vi "GetAngle.vi"(11 "navX Device TypeDef":T1={"navX Interface Protocol"=enum."SPI", "navX Interface Protocol TypeDefs"={"SPIDevRef"={"DevStatus"={"status"=FALSE, "code"=0, "source"=""}, "Handle"=0, "Controller"=enum."Controller 1", "SPI Bus"=enum."SPI On-Board, CS0"}, "I2CDevRef"={"DevStatus"={"status"=FALSE, "code"=0, "source"=""}, "Controller"=enum."Controller 1", "Device Address"=0, "Handle"=0, "I2C Bus"=enum."Invalid"}}, "navX System Information"={"Board Information"={"WhoAmI (50 | 0x32)"=0, "Board Revision"=0, "Firmware Major Version"=0, "Firmware Minor Version"=0, "NAVX_BOARD_CAPABILITY"={"OMNIMOUNT"=FALSE, "YAW_RESET"=FALSE, "VEL_AND_DISP"=FALSE}, "NAVX_BOARD_YAW_AXIS"={"BOARD_YAW_AXIS_UP"=FALSE, "BOARD_YAW_AXIS"=0}}, "Status"={"Update Rate Hz"=0, "Accelerometer Full-Scale Range"=0, "Gyro Full-Scale Range"=0, "NAVX_OP_STATUS"=0, "NAVX_CAL_STATUS"=0, "NAVX_SELFTEST_STATUS"=0, "NAVX_SENSOR_STATUS"={"MOVING"=FALSE, "YAW_STABLE"=FALSE, "MAG_DISTURBANCE"=FALSE, "ALTITUDE_VALID"=FALSE, "SEALEVEL_PRESS_SET"=FALSE, "FUSED_HEADING_VALID"=FALSE}}, "Offsets"={"Yaw"=0.0, "Quat W"=0.0, "Quat X"=0.0, "Quat Y"=0.0, "Quat Z"=0.0}, "LastSampleTimestamp"=0.0, "LastSampleValid"=FALSE, "LastSampleValidTimestamp"=0.0}, "navX Common Information"={"Update Rate (4Hz-60Hz)"=50, "refnum name"="", "error"={"status"=FALSE, "code"=0, "source"=""}, "LastSampleFPGATimestamp"=0.0}} {"navX Common Information"."Update Rate (4Hz-60Hz)" min=4 max=60 step=1; "navX System Information"."Status"."NAVX_OP_STATUS" items=["INITIALIZING", "SELFTEST_IN_PROGRESS", "ERROR", "IMU_AUTOCAL_IN_PROGRESS", "NORMAL"]; "navX System Information"."Status"."NAVX_CAL_STATUS" items=["IMU_CAL_STATE_MASK"=3, "IMU_CAL_INPROGRESS"=0, "IMU_CAL_ACCUMULATE"=1, "IMU_CAL_COMPLETE"=2, "MAG_CAL_COMPLETE"=4, "BARO_CAL_COMPLETE"=8]; "navX Interface Protocol TypeDefs"."I2CDevRef"."Device Address" format="%.0x"}) -> (1 "Valid?":bool, 2 "ContinuousAngle":dbl, 3 "navX Device TypeDef":T1={"navX Interface Protocol"=enum."SPI", "navX Interface Protocol TypeDefs"={"SPIDevRef"={"DevStatus"={"status"=FALSE, "code"=0, "source"=""}, "Handle"=0, "Controller"=enum."Controller 1", "SPI Bus"=enum."SPI On-Board, CS0"}, "I2CDevRef"={"DevStatus"={"status"=FALSE, "code"=0, "source"=""}, "Controller"=enum."Controller 1", "Device Address"=0, "Handle"=0, "I2C Bus"=enum."Invalid"}}, "navX System Information"={"Board Information"={"WhoAmI (50 | 0x32)"=0, "Board Revision"=0, "Firmware Major Version"=0, "Firmware Minor Version"=0, "NAVX_BOARD_CAPABILITY"={"OMNIMOUNT"=FALSE, "YAW_RESET"=FALSE, "VEL_AND_DISP"=FALSE}, "NAVX_BOARD_YAW_AXIS"={"BOARD_YAW_AXIS_UP"=FALSE, "BOARD_YAW_AXIS"=0}}, "Status"={"Update Rate Hz"=0, "Accelerometer Full-Scale Range"=0, "Gyro Full-Scale Range"=0, "NAVX_OP_STATUS"=0, "NAVX_CAL_STATUS"=0, "NAVX_SELFTEST_STATUS"=0, "NAVX_SENSOR_STATUS"={"MOVING"=FALSE, "YAW_STABLE"=FALSE, "MAG_DISTURBANCE"=FALSE, "ALTITUDE_VALID"=FALSE, "SEALEVEL_PRESS_SET"=FALSE, "FUSED_HEADING_VALID"=FALSE}}, "Offsets"={"Yaw"=0.0, "Quat W"=0.0, "Quat X"=0.0, "Quat Y"=0.0, "Quat Z"=0.0}, "LastSampleTimestamp"=0.0, "LastSampleValid"=FALSE, "LastSampleValidTimestamp"=0.0}, "navX Common Information"={"Update Rate (4Hz-60Hz)"=50, "refnum name"="", "error"={"status"=FALSE, "code"=0, "source"=""}, "LastSampleFPGATimestamp"=0.0}} {"navX Common Information"."Update Rate (4Hz-60Hz)" min=4 max=60 step=1; "navX System Information"."Status"."NAVX_OP_STATUS" items=["INITIALIZING", "SELFTEST_IN_PROGRESS", "ERROR", "IMU_AUTOCAL_IN_PROGRESS", "NORMAL"]; "navX System Information"."Status"."NAVX_CAL_STATUS" items=["IMU_CAL_STATE_MASK"=3, "IMU_CAL_INPROGRESS"=0, "IMU_CAL_ACCUMULATE"=1, "IMU_CAL_COMPLETE"=2, "MAG_CAL_COMPLETE"=4, "BARO_CAL_COMPLETE"=8]; "navX Interface Protocol TypeDefs"."I2CDevRef"."Device Address" format="%.0x"})   [LabVIEW 2014, in "navX-MXP IMU.lvlib"]
doc: "Returns the angle, in degrees, from the original heading that the robot is currently facing.\n\nNote that this angle is continuous (meaning that it can return values greater than 360 degrees and less than -360 degrees. You can devide by 360 and use the remainder to yield an angle with a value from -360 to 360 degrees.\n\nThis VI is created to provide an interface which is compatible with the WPI LabVIEW Library GetAngle.vi ."
uses:
  navX-MXP IMU.lvlib
  TypeDefs/navX Device TypeDef.ctl
  TypeDefs/Value TypeDefs/navX Interface Protocol.ctl
  <vilib>/Rock Robotics/WPI/SPI/WPI_SPIDevRef.ctl
  <vilib>/Rock Robotics/SystemInterfaces/Typedef/FPGA_TypedefDigitalModule.ctl
  <vilib>/Rock Robotics/SystemInterfaces/spilib/spi_bus.ctl
  <vilib>/Rock Robotics/WPI/I2C/WPI_I2CDevRef.ctl
  <vilib>/Rock Robotics/SystemInterfaces/i2clib/i2c_bus.ctl
  TypeDefs/Data TypeDefs/navX Board Information.ctl
  TypeDefs/Value TypeDefs/navX NAVX_BOARD_CAPABILITY.ctl
  TypeDefs/Value TypeDefs/navX NAVX_BOARD_YAW_AXIS.ctl
  TypeDefs/Data TypeDefs/navX Status Data.ctl
  TypeDefs/Value TypeDefs/navX NAVX_OP_STATUS.ctl
  TypeDefs/Value TypeDefs/navX NAVX_CAL_STATUS.ctl
  TypeDefs/Value TypeDefs/navX NAVX_SENSOR_STATUS.ctl
  TypeDefs/Data TypeDefs/navX Offsets Data.ctl
  TypeDefs/Value TypeDefs/navX Update Rate.ctl
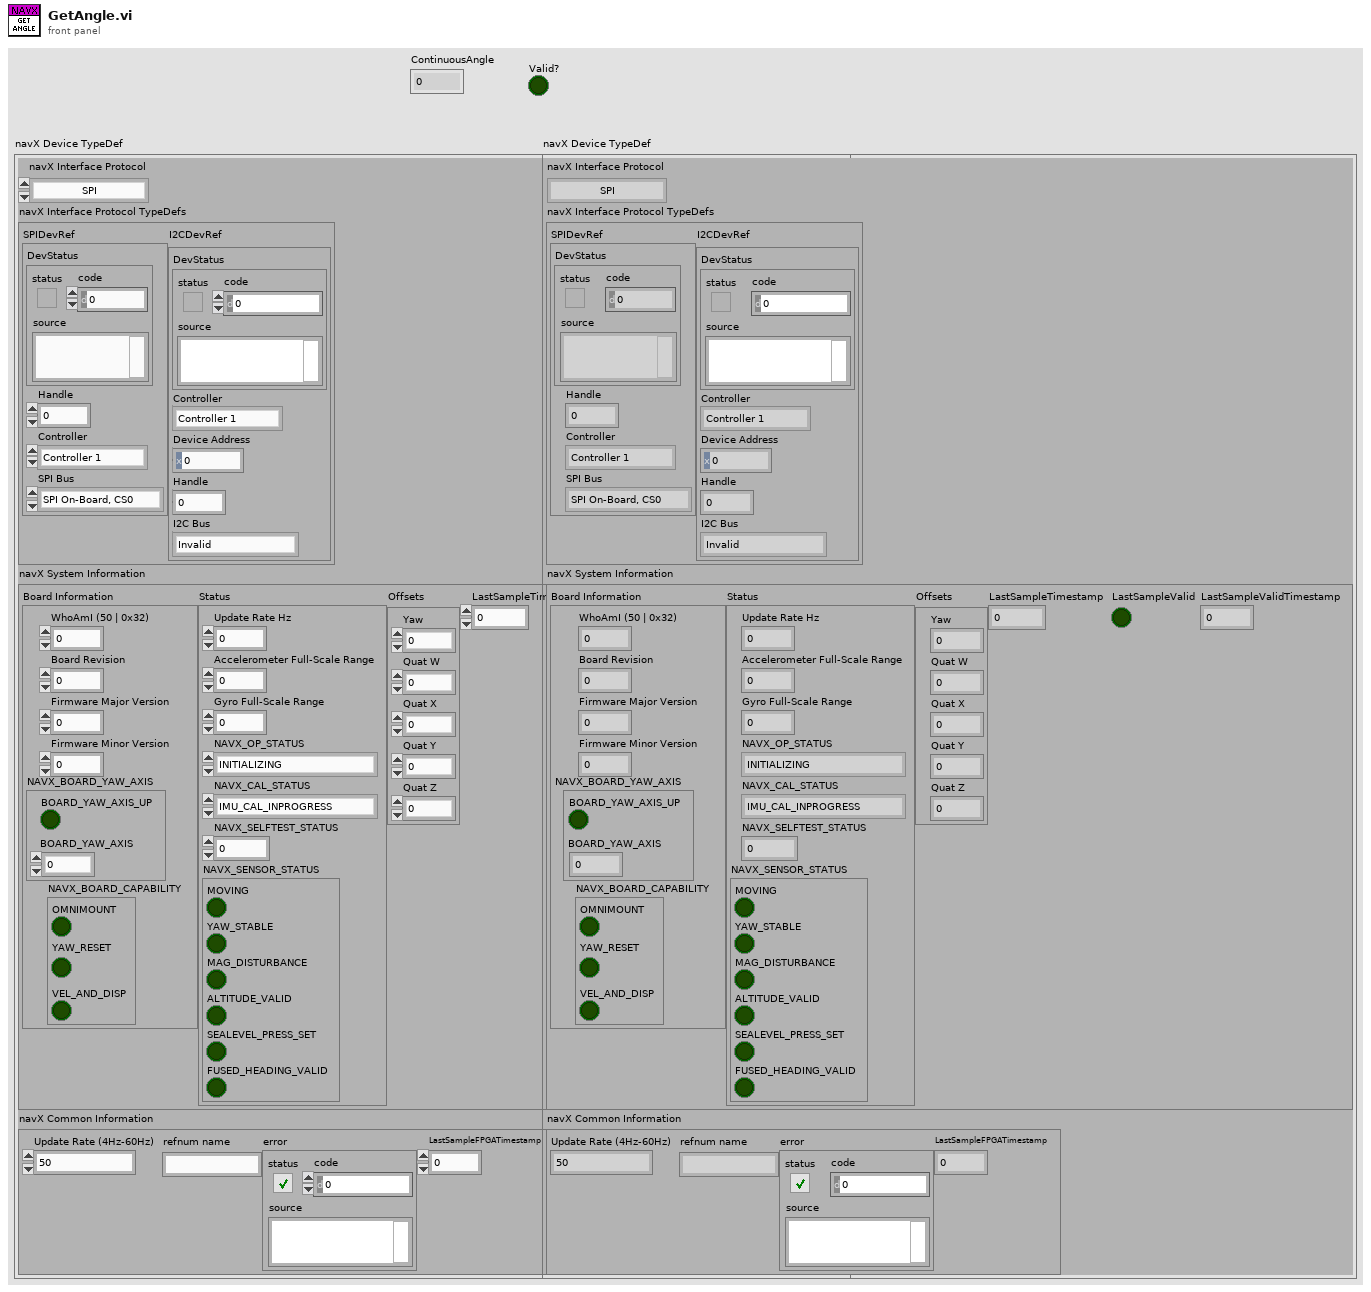
[diagram p1: front panel]
types:
  T1 = typedef "navX-MXP IMU.lvlib/navX Device TypeDef.ctl" = cluster{"navX Interface Protocol":T2, "navX Interface Protocol TypeDefs":cluster{"SPIDevRef":T3, "I2CDevRef":T6}, "navX System Information":cluster{"Board Information":T8, "Status":T11, "Offsets":T15, "LastSampleTimestamp":dbl, "LastSampleValid":bool, "LastSampleValidTimestamp":dbl}, "navX Common Information":cluster{"Update Rate (4Hz-60Hz)":T16, "refnum name":string, "error":errorcluster, "LastSampleFPGATimestamp":dbl}}
  T2 = typedef "navX-MXP IMU.lvlib/navX Interface Protocol.ctl" = enum16{"SPI", "I2C", "SERIAL"}
  T3 = typedef "WPI_SPIDevRef.ctl" = cluster{"DevStatus":errorcluster, "Handle":i32, "Controller":T4, "SPI Bus":T5}
  T4 = typedef "FPGA_TypedefDigitalModule.ctl" = enum16{"Controller 1"}
  T5 = typedef "spi_bus.ctl" = enum16{"SPI On-Board, CS0", "SPI On-Board, CS1", "SPI On-Board, CS2", "SPI On-Board, CS3", "SPI MXP", "Invalid"}
  T6 = typedef "WPI_I2CDevRef.ctl" = cluster{"DevStatus":errorcluster, "Controller":T4, "Device Address":u8, "Handle":i32, "I2C Bus":T7}
  T7 = typedef "i2c_bus.ctl" = enum16{"I2C On-Board", "I2C MXP", "Invalid"}
  T8 = typedef "navX-MXP IMU.lvlib/navX Board Information.ctl" = cluster{"WhoAmI (50 | 0x32)":u8, "Board Revision":u8, "Firmware Major Version":u8, "Firmware Minor Version":u8, "NAVX_BOARD_CAPABILITY":T9, "NAVX_BOARD_YAW_AXIS":T10}
  T9 = typedef "navX-MXP IMU.lvlib/navX NAVX_BOARD_CAPABILITY.ctl" = cluster{"OMNIMOUNT":bool, "YAW_RESET":bool, "VEL_AND_DISP":bool}
  T10 = typedef "navX-MXP IMU.lvlib/navX NAVX_BOARD_YAW_AXIS.ctl" = cluster{"BOARD_YAW_AXIS_UP":bool, "BOARD_YAW_AXIS":u8}
  T11 = typedef "navX-MXP IMU.lvlib/navX Status Data.ctl" = cluster{"Update Rate Hz":u8, "Accelerometer Full-Scale Range":u8, "Gyro Full-Scale Range":u16, "NAVX_OP_STATUS":T12, "NAVX_CAL_STATUS":T13, "NAVX_SELFTEST_STATUS":u8, "NAVX_SENSOR_STATUS":T14}
  T12 = typedef "navX-MXP IMU.lvlib/navX NAVX_OP_STATUS.ctl" = u8
  T13 = typedef "navX-MXP IMU.lvlib/navX NAVX_CAL_STATUS.ctl" = u8
  T14 = typedef "navX-MXP IMU.lvlib/navX NAVX_SENSOR_STATUS.ctl" = cluster{"MOVING":bool, "YAW_STABLE":bool, "MAG_DISTURBANCE":bool, "ALTITUDE_VALID":bool, "SEALEVEL_PRESS_SET":bool, "FUSED_HEADING_VALID":bool}
  T15 = typedef "navX-MXP IMU.lvlib/navX Offsets Data.ctl" = cluster{"Yaw":dbl, "Quat W":dbl, "Quat X":dbl, "Quat Y":dbl, "Quat Z":dbl}
  T16 = typedef "navX-MXP IMU.lvlib/navX Update Rate.ctl" = u8
  T17 = typedef "navX-MXP IMU.lvlib/navX YPRH Data.ctl" = cluster{"Yaw":dbl, "Pitch":dbl, "Roll":dbl, "Heading":dbl}
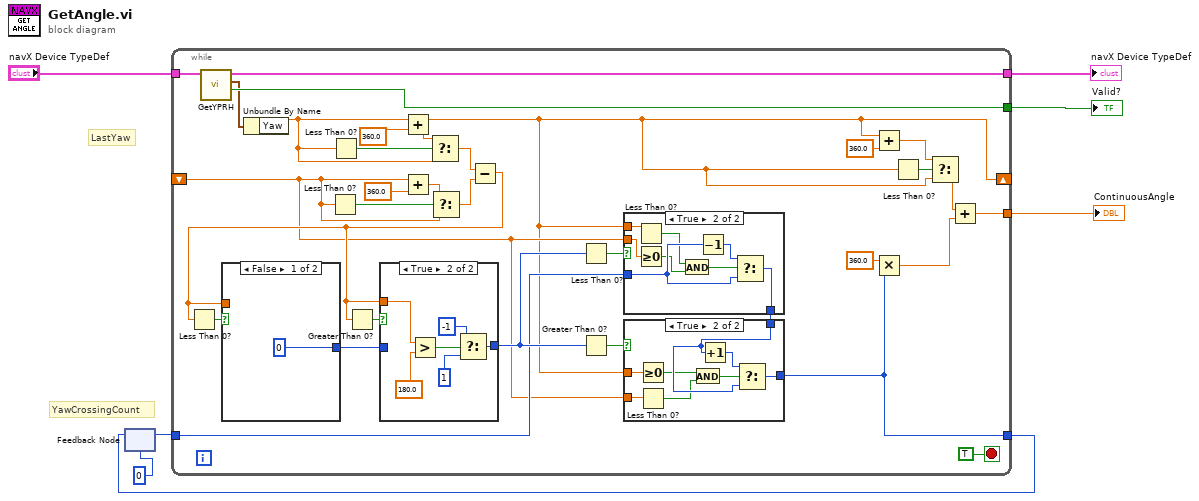
[diagram p0: block diagram]
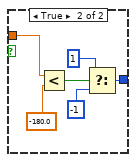
[diagram p5: hidden frame]
diagram:
  # "YawCrossingCount"
  # "LastYaw"
  n1 = feedback #1(0) -> (w3:i32)
  n2 = while {
    shift-right: [w9] -> _
    shift-left: _ -> [w10]
    tunnel: [w38] -> w5
    tunnel: "navX Device TypeDef" -> [w35]
    tunnel: [w34] -> w6
    tunnel: [w24] -> w4
    tunnel: w3 -> [w22]
    tunnel: [w21] -> w1
    stop <- TRUE stop-if-true
    n3 = call "GetYPRH.vi"("navX Device TypeDef"=w35) -> ("Valid?"=w38:bool, "YPRH"=w33:T17, "navX Device TypeDef"=w34:T1)  [unwired: 8 in]
    n4 = Unbundle By Name(w33) -> ("Yaw"=w9:dbl)
    n5 = Less Than 0?(x=w10) -> (x < 0?=w14:bool)
    n6 = Less Than 0?(x=w9) -> (x < 0?=w15:bool)
    n7 = Add(x=w9, y=360.0) -> (x+y=w8:dbl)
    n8 = Add(x=w10, y=360.0) -> (x+y=w11:dbl)
    n9 = Select(t=w8, s=w15, f=w9) -> (s? t:f=w13:dbl)
    n10 = Select(t=w11, s=w14, f=w10) -> (s? t:f=w12:dbl)
    n11 = Subtract(x=w13, y=w12) -> (x-y=w16:dbl)
    n12 = Less Than 0?(x=w16) -> (x < 0?=w18:bool)
    n13 = case shown="False" w18 {
      tunnel: [0 w67] -> w32
      tunnel: w16 -> [_ w66]
      frame False {
      }
      frame True {
        n14 = Less?(x=w66, y=-180.0) -> (x < y?=w70:bool)
        n15 = Select(t=1, s=w70, f=-1) -> (s? t:f=w67:i32)
      }
    }
    n16 = Greater Than 0?(x=w16) -> (x > 0?=w17:bool)
    n17 = case shown="True" w17 {
      tunnel: [w58 w60] -> w29
      tunnel: w32 -> [w58 _]
      tunnel: w16 -> [_ w59]
      frame False {
      }
      frame True {
        n18 = Greater?(x=w59, y=180.0) -> (0:w63:bool)
        n19 = Select(t=-1, s=w63, f=1) -> (s? t:f=w60:i32)
      }
    }
    n20 = Less Than 0?(x=w29) -> (x < 0?=w31:bool)
    n21 = Greater Than 0?(x=w29) -> (x > 0?=w30:bool)
    n22 = case shown="True" w31 {
      tunnel: w22 -> [w49 w56]
      tunnel: w9 -> [_ w54]
      tunnel: [w49 w55] -> w23
      tunnel: w10 -> [_ w53]
      frame False {
      }
      frame True {
        n23 = Less Than 0?(x=w54) -> (x < 0?=w52:bool)
        n24 = Greater Or Equal To 0?(x=w53) -> (x >= 0?=w51:bool)
        n25 = And(x=w52, y=w51) -> (x .and. y?=w50:bool)
        n26 = Decrement(x=w56) -> (x-1=w57:i32)
        n27 = Select(t=w57, s=w50, f=w56) -> (s? t:f=w55:i32)
      }
    }
    n28 = case shown="True" w30 {
      tunnel: w9 -> [_ w45]
      tunnel: w23 -> [w40 w47]
      tunnel: [w40 w46] -> w21
      tunnel: w10 -> [_ w44]
      frame False {
      }
      frame True {
        n29 = Greater Or Equal To 0?(x=w45) -> (x >= 0?=w42:bool)
        n30 = Less Than 0?(x=w44) -> (x < 0?=w41:bool)
        n31 = And(x=w42, y=w41) -> (x .and. y?=w43:bool)
        n32 = Increment(x=w47) -> (x+1=w48:i32)
        n33 = Select(t=w48, s=w43, f=w47) -> (s? t:f=w46:i32)
      }
    }
    n34 = Add(x=w9, y=360.0) -> (x+y=w19:dbl)
    n35 = Multiply(x=360.0, y=w21) -> (x*y=w25:dbl)
    n36 = Less Than 0?(x=w9) -> (x < 0?=w28:bool)
    n37 = Select(t=w19, s=w28, f=w9) -> (s? t:f=w27:dbl)
    n38 = Add(x=w27, y=w25) -> (x+y=w24:dbl)
  }
  "Valid?" <- w5
  "navX Device TypeDef" <- w6
  "ContinuousAngle" <- w4
  n39 = feedback-in #1(w1) -> ()
